vi "Initialize-message-queues.vi"(8 "error in (no error)":errorcluster, 11 "Object ref in":T1) -> (0 "error out":errorcluster, 3 "Object ref out":T1)   [LabVIEW 2013, in "PowderDeposition.lvlib" / "PD-Main.lvclass"]
uses:
  PD-Main.lvclass
  Object-reference.ctl
  Execution-actions.ctl
  PD-actions.ctl
  PD-Main.lvclass/PD-Main.ctl
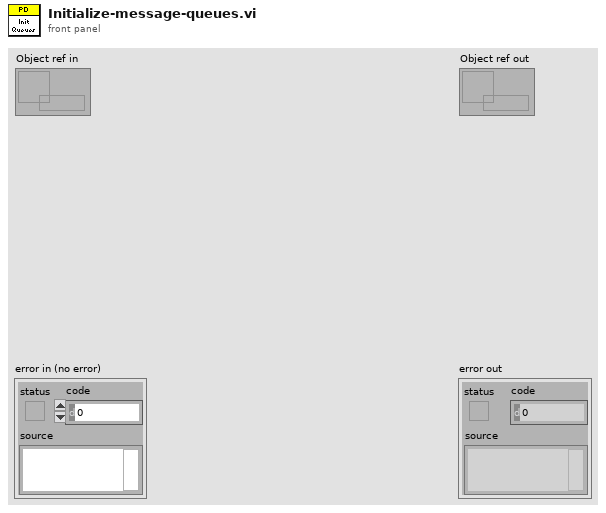
[diagram p1: front panel]
types:
  T1 = typedef "PowderDeposition.lvlib/PD-Main.lvclass/Object-reference.ctl" = refnum<data-value>
  T2 = typedef "PowderDeposition.lvlib/PD-Main.lvclass/PD-actions.ctl" = enum16{"Idle", "Initialize", "Signal initialized", "Activate all motors", "Deactivate all motors", "Update motor activity", "Update selected motor", "Update motor status", "Update selected sequence", "Load sequences with dialog", "Load sequences from file", "Save sequences", "Add to sequence", "Remove from sequence", "Clear sequences", "Update available actions", "Create action", "Edit action", "Execute action", "Execute sequences", "Execute seq with assert", "Abort", "Exit"}
  T3 = typedef "PowderDeposition.lvlib/PD-Main.lvclass/Execution-actions.ctl" = enum16{"Idle", "Execute action", "Execute sequence", "Execute seq with assert", "Exit"}
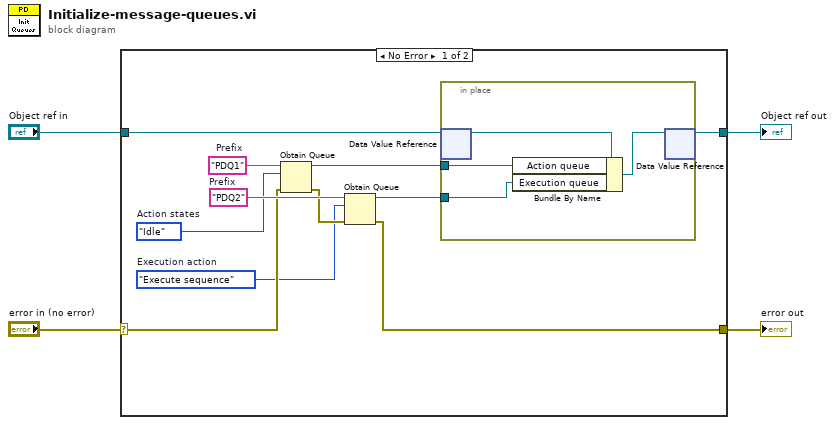
[diagram p0: block diagram]
diagram:
  n1 = case shown="No Error" "error in (no error)" {
    selector: "error in (no error)" -> [w10 w21]
    tunnel: [w8 w21] -> w3
    tunnel: [w14 w20] -> w1
    tunnel: "Object ref in" -> [w15 w20]
    frame No Error {
      w5 = PD-actions."Idle"  # Action states
      w6 = Execution-actions."Execute sequence"  # Execution action
      w12 = "PDQ2"  # Prefix
      w11 = "PDQ1"  # Prefix
      n2 = Obtain Queue(name (unnamed)=w11, element data type=w5, error in (no error)=w10) -> (queue out=w7:refnum<queue>, error out=w9:errorcluster)  [unwired: 2 in, 1 out]
      n3 = Obtain Queue(name (unnamed)=w12, element data type=w6, error in (no error)=w9) -> (queue out=w13:refnum<queue>, error out=w8:errorcluster)  [unwired: 2 in, 1 out]
      n4 = in-place {
        in-place-border: w7 -> [w17]
        in-place-border: w13 -> [w16]
        n5 = in-place-dvr #1(w15) -> (w19:refnum<class "PD-Main.lvclass">)  [unwired: 1 out]
        n6 = Bundle By Name(cluster=w19, "Action queue"=w17, "Execution queue"=w16) -> (w18:refnum<class "PD-Main.lvclass">)
        n7 = in-place-dvr #1(w18) -> (w14:T1)  [unwired: 1 out]
      }
    }
    frame Error {
    }
  }
  "error out" <- w3
  "Object ref out" <- w1
